vi "Build Graph.vi"(10 "Temperature Array":dbl[](array[numeric]), 11 "Time Array":dbl[](array[numeric])) -> (3 "XY Graph":cluster{"X":dbl, "Y":dbl}[](array[cluster]))   [LabVIEW 2016]
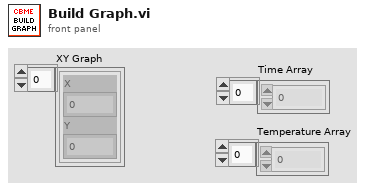
[diagram p1: front panel]
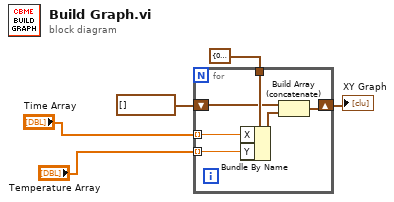
[diagram p0: block diagram]
diagram:
  n1 = for {
    shift-right: [w8] -> w5
    shift-left: cluster{"X":dbl, "Y":dbl}[] [] ("XY Graph") -> [w9]
    tunnel: cluster{"X":dbl, "Y":dbl} {"X"=0.0, "Y"=0.0} -> [w11]
    tunnel: "Time Array" -> [w7] mode=indexing
    tunnel: "Temperature Array" -> [w6] mode=indexing
    n2 = Bundle By Name(cluster=w11, "X"=w7, "Y"=w6) -> (w10:cluster{"X":dbl, "Y":dbl})
    n3 = Build Array (concatenate)(w9, w10) -> (w8:cluster{"X":dbl, "Y":dbl}[])
  }
  "XY Graph" <- w5
